vi "Reset MPU9250 SPI.vi"(5 "CS":refnum<class "SPI CS.lvclass">, 7 "SPI":refnum<class "SPI.lvclass">, 8 "error in (no error)":errorcluster, 11 "Session In":refnum<class "Session.lvclass">) -> (0 "error out":errorcluster={"status"=TRUE, "code"=-1073807346, "source"="Property Node (arg 1) in CTI-Visa.lvlib:Check Previous Error.vi->CTI-Visa.lvlib:Set Digital Output.vi->CTI-Visa-DeviceLib.lvlib:Reset MPU9250 SPI.vi"}, 3 "Session Out":refnum<class "Session.lvclass">)   [LabVIEW 2020, in "CTI-Visa-DeviceLib.lvlib"]
uses:
  CTI-Visa-DeviceLib.lvlib
  CTI/SPI/SPI.lvclass
  CTI/Session/Session.lvclass
  CTI/SPI CS/SPI CS.lvclass
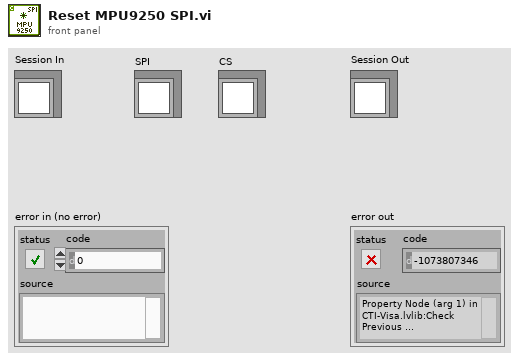
[diagram p1: front panel]
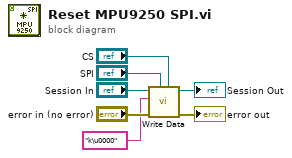
[diagram p0: block diagram]
diagram:
  n1 = call "Write Data.vi"("CS (None)"="CS", "SPI"="SPI", "error in (no error)"="error in (no error)", "Data"="k\u0000", "Session In"="Session In") -> ("error out"=→"error out":errorcluster, "Session Out"=→"Session Out":refnum<class "Session.lvclass">)  [unwired: 5 in]
